vi "Slow Fibonacci.vi"(1 "n":u32) -> (0 "Fibonacci(n)":u32)   [LabVIEW 2018]
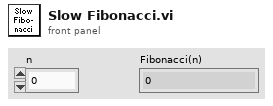
[diagram p1: front panel]
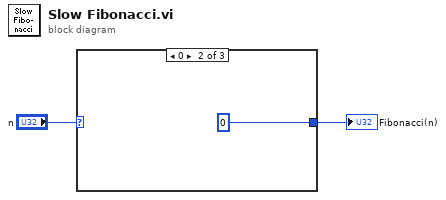
[diagram p0: block diagram]
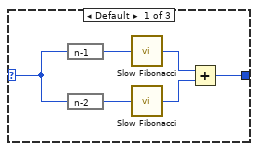
[diagram p2: hidden frame]
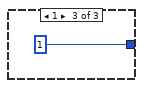
[diagram p3: hidden frame]
diagram:
  n1 = case shown="0" "n" {
    selector: "n" -> [w8 _ _]
    tunnel: [w3 u32 0 ("Fibonacci(n)") u32 1 ("Fibonacci(n)")] -> w1
    frame Default {
      n2 = expression code="n-1"(w8) -> (w6:u32)
      n3 = expression code="n-2"(w8) -> (w7:u32)
      n4 = call "Slow Fibonacci.vi"("n"=w6) -> ("Fibonacci(n)"=w5:u32)
      n5 = call "Slow Fibonacci.vi"("n"=w7) -> ("Fibonacci(n)"=w4:u32)
      n6 = Add(x=w5, y=w4) -> (x+y=w3:u32)
    }
    frame 0 {
    }
    frame 1 {
    }
  }
  "Fibonacci(n)" <- w1
